vi "pumonarytesting_works.vi"() -> ()   [LabVIEW 2014]
uses:
  <vilib>/vision/NI_Vision_Development_Module.lvlib
  <instrlib>/KD Scientific 2XX Series/KD Scientific 2XX Series.lvlib
panel:
  in  "Number of Cycles":i32
  in  "Min Pressure":dbl
  in  "Max Pressure":dbl
  out "Status":T1
  in  "stop 2":bool
  out "Delivered Volume":dbl
  out "Units":string
  in  "Baud Rate (9600)":u32(ring)=9600 items=["300"=300, "1200"=1200, "2400"=2400, "4800"=4800, "9600"=9600]
  in  "Withdrawal Settings":T2={"Flow Rate (5)"=5.0, "Volume (10)"=10.0, "Volume Units (ml)"=enum."milliliters (ml)", "Rate Units (ml/min.)"=enum."milliliters per minute (ml/min.)"} {"Volume (10)" format="%#.3g"}
  in  "Diameter (8.75 mm)":dbl=8.75
  in  "Infusion Settings":T2={"Flow Rate (5)"=5.0, "Volume (10)"=10.0, "Volume Units (ml)"=enum."milliliters (ml)", "Rate Units (ml/min.)"=enum."milliliters per minute (ml/min.)"}
  in  "Address (0)":i32 format="%0.0f"
  in  "error in (no error)":errorcluster
  in  "VISA resource name":refnum<visa-resource-name>="COM1"
  in  "stop 4":bool
  in  "stop":bool
  out "Image":T3(plugin-control)
  out "Particle Measurements (Pixels) (Particle Analysis 1)":dbl[][](array[numeric]) format="%.2f"
  out "subarray":dbl[](array[numeric])
  out "The diameter":dbl[](array[numeric])
  in  "stop (F)":bool
  out "Data from Transducer":dynamicdata(graph) caption="Voltage from Transducer V"
  out "Voltage from pressure transducer":dbl[](array[numeric])
  out "Pressure mm Hg":dbl[](graph)
  in  "Calibration factor":dbl[](array[numeric])
  in  "Zero Error":dbl[](array[numeric])
  out "pressure mm Hg":dbl[](array[numeric])
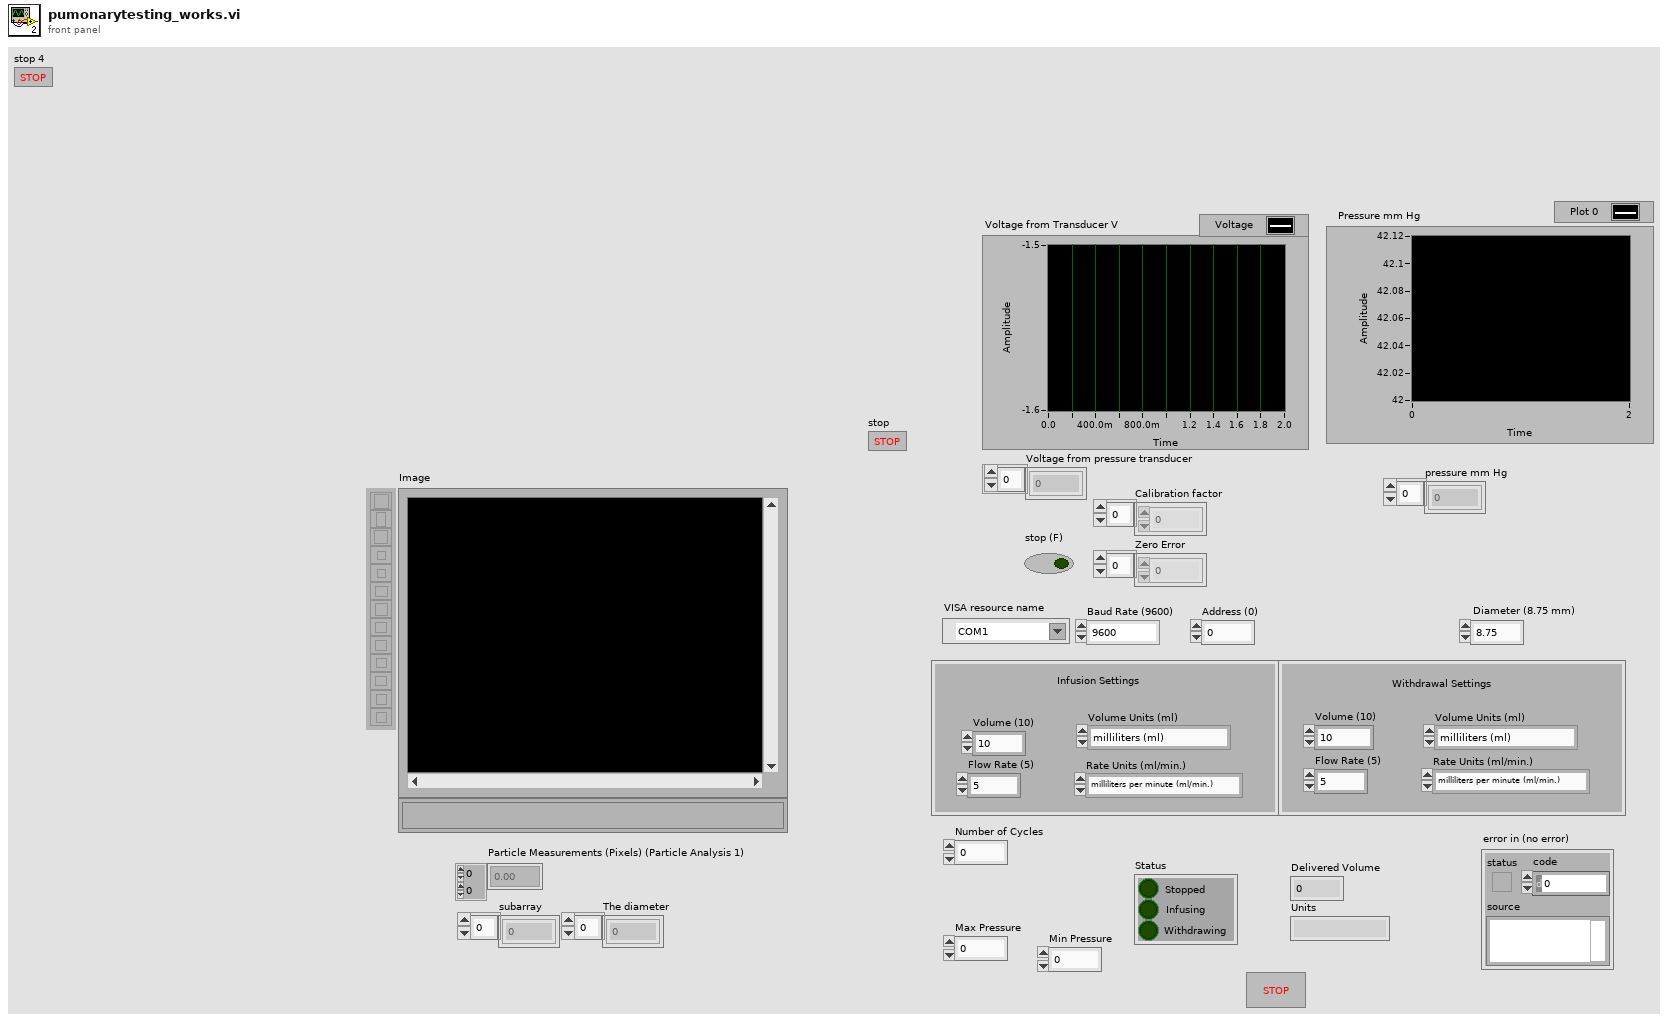
[diagram p1: front panel]
types:
  T1 = cluster{"Stopped":bool, "Infusing":bool, "Withdrawing":bool}
  T2 = cluster{"Flow Rate (5)":dbl, "Volume (10)":dbl, "Volume Units (ml)":enum16{"milliliters (ml)", "microliters (ul)"}, "Rate Units (ml/min.)":enum16{"milliliters per minute (ml/min.)", "milliliters per hour (ml/hr.)", "microliters per minute (ul/min.)", "microliters per hour (ul/hr.)"}}
  T3 = typedef "IMAQ Image.ctl" = refnum<image>
  T4 = typedef "Board Id" = u8
  T5 = typedef "ROI Descriptor" = cluster{"Global Rectangle":i32[], "Contours":cluster{"ID":enum32{"External", "Internal"}, "Type":u32, "Coordinates":i32[]}[]}
  T6 = enum16{"milliliters per minute (ml/min.)", "milliliters per hour (ml/hr.)", "microliters per minute (ul/min.)", "microliters per hour (ul/hr.)"}
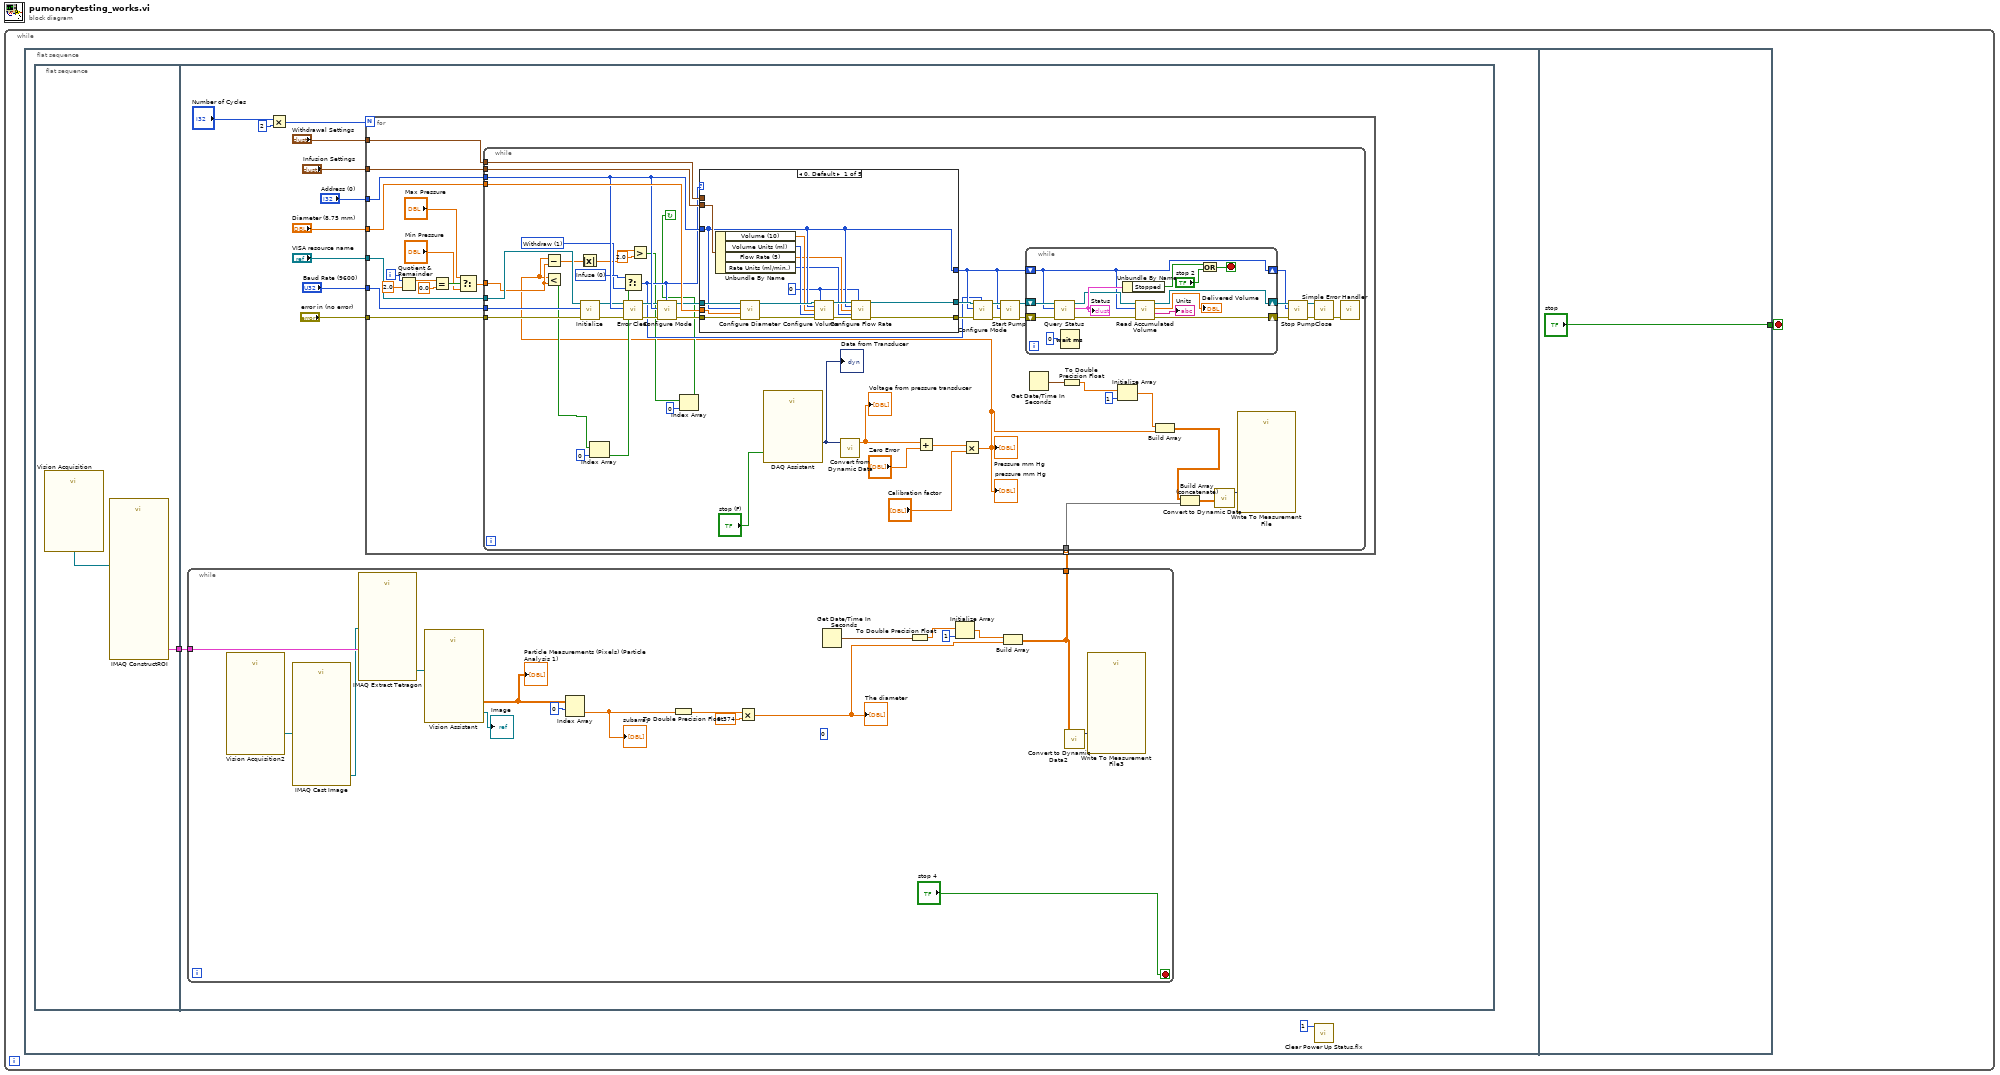
[diagram p0: block diagram]
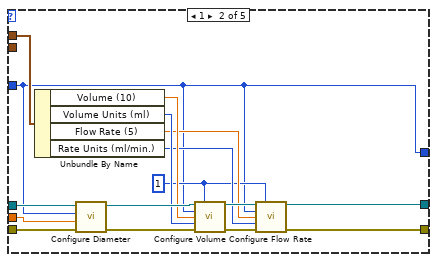
[diagram p2: hidden frame]
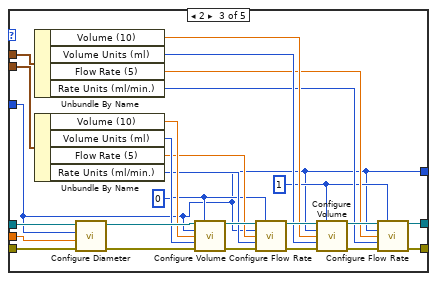
[diagram p3: hidden frame]
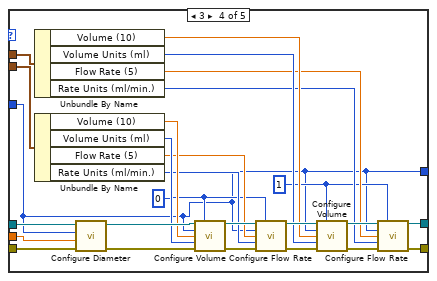
[diagram p4: hidden frame]
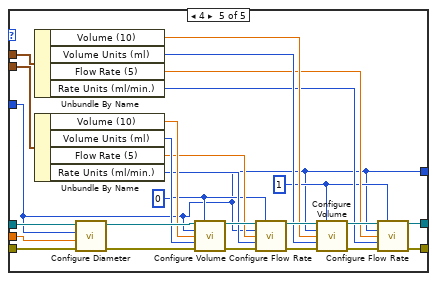
[diagram p5: hidden frame]
diagram:
  n1 = while {
    stop <- w1 stop-if-true
    n2 = flat-sequence {
      tunnel: ["stop"] -> w1
      frame #0 {
        n3 = flat-sequence {
          tunnel: [w4] -> w3
          tunnel: w3 -> [w17]
          frame #0 {
            n4 = call "Vision Acquisition"() -> ("Image Out"=w5:T3)  [unwired: 26 in, 1 out]
            n5 = call "IMAQ ConstructROI"("Image"=w5) -> ("ROI Descriptor Out"=w4:T5)  [unwired: 7 in, 3 out]
          }
          frame #1 {
            n6 = while {
              tunnel: w17 -> [w229]
              tunnel: [w212] -> w6
              stop <- "stop 4" stop-if-true
              (unwired) 0 ("index")
              n7 = call "Vision Acquisition2"() -> ("Image Out"=w220:T3)  [unwired: 25 in, 2 out]
              n8 = call "IMAQ Cast Image"("Image Src"=w220) -> ("Image Dst Out"=w226:T3)  [unwired: 9 in, 1 out]
              n9 = call-poly "IMAQ Extract Tetragon"("ROI Descriptor"=w229, "Image Src"=w226) -> ("Image Dst Out"=w227:T3)  [unwired: 8 in, 1 out]
              n10 = call "Vision Assistant"("Image In"=w227) -> ("Image Out"=→"Image":T3, "Particle Measurements (Pixels) (Particle Analysis 1)"=w225:dbl[][])  [unwired: 23 in, 2 out]
              "Particle Measurements (Pixels) (Particle Analysis 1)" <- w225
              n11 = Index Array(array=w225, index (row)=0) -> (element=w223:dbl[])  [unwired: 1 in]
              "subarray" <- w223
              n12 = To Double Precision Float(number=w223) -> (double precision float=w222:dbl[])
              n13 = Multiply(x=w222, y=0.374) -> (x*y=w214:dbl[])
              "The diameter" <- w214
              n14 = Get Date/Time In Seconds() -> (seconds since 1Jan1904=w218:timestamp)
              n15 = To Double Precision Float(number=w218) -> (double precision float=w217:dbl)
              n16 = Initialize Array(w217, 1 ("dimension size")) -> (w215:dbl[])
              n17 = Build Array(w215, w214) -> (w212:dbl[][])
              n18 = call "Convert to Dynamic Data2"("2D Array"=w212) -> ("Dynamic Data Type"=w213:dynamicdata)  [unwired: 3 in]
              n19 = call "Write To Measurement File3"("Signals"=w213) -> ()  [unwired: 16 in, 3 out]
            }
            n20 = Multiply(x="Number of Cycles", y=2) -> (x*y=w16:i32)
            n21 = for {
              N: w16 -> [_]
              tunnel: "VISA resource name" -> [w33]
              tunnel: "error in (no error)" -> [w32]
              tunnel: "Infusion Settings" -> [w31]
              tunnel: "Withdrawal Settings" -> [w30]
              tunnel: "Diameter (8.75 mm)" -> [w29]
              tunnel: "Baud Rate (9600)" -> [w28]
              tunnel: "Address (0)" -> [w27]
              tunnel: w6 -> [w18] mode=indexing
              i -> [w25]
              n22 = Quotient & Remainder(x=w25, y=2.0) -> (x-y*floor(x/y)=w23:dbl)  [unwired: 1 out]
              n23 = Equal?(x=w23, y=0.0) -> (x = y?=w22:bool)
              n24 = Select(t="Max Pressure", s=w22, f="Min Pressure") -> (s? t:f=w19:dbl)
              n25 = while {
                tunnel: w33 -> [w87]
                tunnel: w32 -> [w86]
                tunnel: w31 -> [w85]
                tunnel: w30 -> [w84]
                tunnel: w29 -> [w83]
                tunnel: w28 -> [w82]
                tunnel: w27 -> [w81]
                tunnel: w19 -> [w58]
                tunnel: w18 -> [w37]
                stop <- w43 continue-if-true
                w60 = u16 1 items=["Withdraw"=1]
                w61 = u16 0 items=["Infuse"] ("Mode (infuse)")
                n26 = call <instrlib>:"Initialize.vi"("error in (no error)"=w86, "Baud Rate (9600)"=w82, "VISA resource name"=w87) -> ("error out"=w63:errorcluster, "VISA resource name out"=w62:refnum<visa-resource-name>)  [unwired: 7 in]
                n27 = call <instrlib>:"Error Clear.vi"("error in (no error)"=w63, "Address (0)"=w81, "VISA resource name"=w62) -> ("error out"=w64:errorcluster, "VISA resource name out"=w65:refnum<visa-resource-name>)  [unwired: 6 in, 1 out]
                n28 = call "DAQ Assistant"("stop (T)"="stop (F)") -> ("data"=w49:dynamicdata)  [unwired: 16 in, 2 out]
                "Data from Transducer" <- w49
                n29 = call "Convert from Dynamic Data"("Dynamic Data Type"=w49) -> ("Array"=w52:dbl[])  [unwired: 3 in]
                "Voltage from pressure transducer" <- w52
                n30 = Add(x=w52, y="Zero Error") -> (x+y=w50:dbl[])
                n31 = Multiply(x=w50, y="Calibration factor") -> (x*y=w38:dbl[])
                "Pressure mm Hg" <- w38
                "pressure mm Hg" <- w38
                n32 = Subtract(x=w38, y=w58) -> (x-y=w57:dbl[])
                n33 = Less?(x=w38, y=w58) -> (x < y?=w48:bool[])
                n34 = Absolute Value(x=w57) -> (abs(x)=w56:dbl[])
                n35 = Index Array(array=w48, index=0) -> (element=w46:bool)
                n36 = Select(t=w61, s=w46, f=w60) -> (s? t:f=w59:u16)
                n37 = Greater?(x=w56, y=2.0) -> (0:w45:bool[])
                n38 = call <instrlib>:"Configure Mode.vi"("Mode (infuse)"=w59, "error in (no error)"=w64, "Address (0)"=w81, "VISA resource name"=w65) -> ("error out"=w67:errorcluster, "VISA resource name out"=w66:refnum<visa-resource-name>)  [unwired: 6 in]
                n39 = Index Array(array=w45, index=0) -> (element=w43:bool)
                n40 = case shown="0, Default" w59 {
                  tunnel: w85 -> [w97 _ w145 w171 w197]
                  tunnel: w84 -> [_ w119 w144 w170 w196]
                  tunnel: w66 -> [w103 w118 w143 w169 w195]
                  tunnel: w67 -> [w102 w114 w142 w168 w194]
                  tunnel: w83 -> [w96 w110 w125 w151 w177]
                  tunnel: [w95 w104 w120 w146 w172] -> w68
                  tunnel: w81 -> [w95 w104 w120 w146 w172]
                  tunnel: [w90 w115 w122 w148 w174] -> w72
                  tunnel: [w89 w111 w121 w147 w173] -> w71
                  frame 0, Default {
                    w88 = 0
                    n41 = Unbundle By Name(w97) -> ("Volume (10)"=w94:dbl, "Volume Units (ml)"=w93:enum16{"milliliters (ml)", "microliters (ul)"}, "Flow Rate (5)"=w92:dbl, "Rate Units (ml/min.)"=w91:T6)
                    n42 = call <instrlib>:"Configure Diameter.vi"("error in (no error)"=w102, "Diameter (8.75 mm)"=w96, "Address (0)"=w95, "VISA resource name"=w103) -> ("error out"=w100:errorcluster, "VISA resource name out"=w101:refnum<visa-resource-name>)  [unwired: 6 in]
                    n43 = call <instrlib>:"Configure Volume.vi"("VISA resource name"=w101, "Mode (infuse)"=w88, "Address (0)"=w95, "Volume (100)"=w94, "Units (0: milliliters)"=w93, "error in (no error)"=w100) -> ("VISA resource name out"=w99:refnum<visa-resource-name>, "error out"=w98:errorcluster)  [unwired: 8 in]
                    n44 = call <instrlib>:"Configure Flow Rate.vi"("VISA resource name"=w99, "Mode (infuse)"=w88, "Address (0)"=w95, "Flow Rate (5)"=w92, "Units (0: milliliters per minute)"=w91, "error in (no error)"=w98) -> ("VISA resource name out"=w90:refnum<visa-resource-name>, "error out"=w89:errorcluster)  [unwired: 8 in]
                  }
                  frame 1 {
                    w105 = 1
                    n45 = Unbundle By Name(w119) -> ("Volume (10)"=w109:dbl, "Volume Units (ml)"=w108:enum16{"milliliters (ml)", "microliters (ul)"}, "Flow Rate (5)"=w107:dbl, "Rate Units (ml/min.)"=w106:T6)
                    n46 = call <instrlib>:"Configure Diameter.vi"("error in (no error)"=w114, "Diameter (8.75 mm)"=w110, "Address (0)"=w104, "VISA resource name"=w118) -> ("error out"=w113:errorcluster, "VISA resource name out"=w117:refnum<visa-resource-name>)  [unwired: 6 in]
                    n47 = call <instrlib>:"Configure Volume.vi"("VISA resource name"=w117, "Mode (infuse)"=w105, "Address (0)"=w104, "Volume (100)"=w109, "Units (0: milliliters)"=w108, "error in (no error)"=w113) -> ("VISA resource name out"=w116:refnum<visa-resource-name>, "error out"=w112:errorcluster)  [unwired: 8 in]
                    n48 = call <instrlib>:"Configure Flow Rate.vi"("VISA resource name"=w116, "Mode (infuse)"=w105, "Address (0)"=w104, "Flow Rate (5)"=w107, "Units (0: milliliters per minute)"=w106, "error in (no error)"=w112) -> ("VISA resource name out"=w115:refnum<visa-resource-name>, "error out"=w111:errorcluster)  [unwired: 8 in]
                  }
                  frame 2 {
                    w123 = 1
                    w124 = 0
                    n49 = Unbundle By Name(w144) -> ("Volume (10)"=w129:dbl, "Volume Units (ml)"=w128:enum16{"milliliters (ml)", "microliters (ul)"}, "Flow Rate (5)"=w127:dbl, "Rate Units (ml/min.)"=w126:T6)
                    n50 = Unbundle By Name(w145) -> ("Volume (10)"=w133:dbl, "Volume Units (ml)"=w132:enum16{"milliliters (ml)", "microliters (ul)"}, "Flow Rate (5)"=w131:dbl, "Rate Units (ml/min.)"=w130:T6)
                    n51 = call <instrlib>:"Configure Diameter.vi"("error in (no error)"=w142, "Diameter (8.75 mm)"=w125, "Address (0)"=w120, "VISA resource name"=w143) -> ("error out"=w137:errorcluster, "VISA resource name out"=w141:refnum<visa-resource-name>)  [unwired: 6 in]
                    n52 = call <instrlib>:"Configure Volume.vi"("VISA resource name"=w141, "Mode (infuse)"=w124, "Address (0)"=w120, "Volume (100)"=w133, "Units (0: milliliters)"=w132, "error in (no error)"=w137) -> ("VISA resource name out"=w140:refnum<visa-resource-name>, "error out"=w136:errorcluster)  [unwired: 8 in]
                    n53 = call <instrlib>:"Configure Flow Rate.vi"("VISA resource name"=w140, "Mode (infuse)"=w124, "Address (0)"=w120, "Flow Rate (5)"=w131, "Units (0: milliliters per minute)"=w130, "error in (no error)"=w136) -> ("VISA resource name out"=w139:refnum<visa-resource-name>, "error out"=w135:errorcluster)  [unwired: 8 in]
                    n54 = call <instrlib>:"Configure Volume.vi"("VISA resource name"=w139, "Mode (infuse)"=w123, "Address (0)"=w120, "Volume (100)"=w129, "Units (0: milliliters)"=w128, "error in (no error)"=w135) -> ("VISA resource name out"=w138:refnum<visa-resource-name>, "error out"=w134:errorcluster)  [unwired: 8 in]
                    n55 = call <instrlib>:"Configure Flow Rate.vi"("VISA resource name"=w138, "Mode (infuse)"=w123, "Address (0)"=w120, "Flow Rate (5)"=w127, "Units (0: milliliters per minute)"=w126, "error in (no error)"=w134) -> ("VISA resource name out"=w122:refnum<visa-resource-name>, "error out"=w121:errorcluster)  [unwired: 8 in]
                  }
                  frame 3 {
                    w149 = 1
                    w150 = 0
                    n56 = Unbundle By Name(w170) -> ("Volume (10)"=w155:dbl, "Volume Units (ml)"=w154:enum16{"milliliters (ml)", "microliters (ul)"}, "Flow Rate (5)"=w153:dbl, "Rate Units (ml/min.)"=w152:T6)
                    n57 = Unbundle By Name(w171) -> ("Volume (10)"=w159:dbl, "Volume Units (ml)"=w158:enum16{"milliliters (ml)", "microliters (ul)"}, "Flow Rate (5)"=w157:dbl, "Rate Units (ml/min.)"=w156:T6)
                    n58 = call <instrlib>:"Configure Diameter.vi"("error in (no error)"=w168, "Diameter (8.75 mm)"=w151, "Address (0)"=w146, "VISA resource name"=w169) -> ("error out"=w163:errorcluster, "VISA resource name out"=w167:refnum<visa-resource-name>)  [unwired: 6 in]
                    n59 = call <instrlib>:"Configure Volume.vi"("VISA resource name"=w167, "Mode (infuse)"=w150, "Address (0)"=w146, "Volume (100)"=w159, "Units (0: milliliters)"=w158, "error in (no error)"=w163) -> ("VISA resource name out"=w166:refnum<visa-resource-name>, "error out"=w162:errorcluster)  [unwired: 8 in]
                    n60 = call <instrlib>:"Configure Flow Rate.vi"("VISA resource name"=w166, "Mode (infuse)"=w150, "Address (0)"=w146, "Flow Rate (5)"=w157, "Units (0: milliliters per minute)"=w156, "error in (no error)"=w162) -> ("VISA resource name out"=w165:refnum<visa-resource-name>, "error out"=w161:errorcluster)  [unwired: 8 in]
                    n61 = call <instrlib>:"Configure Volume.vi"("VISA resource name"=w165, "Mode (infuse)"=w149, "Address (0)"=w146, "Volume (100)"=w155, "Units (0: milliliters)"=w154, "error in (no error)"=w161) -> ("VISA resource name out"=w164:refnum<visa-resource-name>, "error out"=w160:errorcluster)  [unwired: 8 in]
                    n62 = call <instrlib>:"Configure Flow Rate.vi"("VISA resource name"=w164, "Mode (infuse)"=w149, "Address (0)"=w146, "Flow Rate (5)"=w153, "Units (0: milliliters per minute)"=w152, "error in (no error)"=w160) -> ("VISA resource name out"=w148:refnum<visa-resource-name>, "error out"=w147:errorcluster)  [unwired: 8 in]
                  }
                  frame 4 {
                    w175 = 1
                    w176 = 0
                    n63 = Unbundle By Name(w196) -> ("Volume (10)"=w181:dbl, "Volume Units (ml)"=w180:enum16{"milliliters (ml)", "microliters (ul)"}, "Flow Rate (5)"=w179:dbl, "Rate Units (ml/min.)"=w178:T6)
                    n64 = Unbundle By Name(w197) -> ("Volume (10)"=w185:dbl, "Volume Units (ml)"=w184:enum16{"milliliters (ml)", "microliters (ul)"}, "Flow Rate (5)"=w183:dbl, "Rate Units (ml/min.)"=w182:T6)
                    n65 = call <instrlib>:"Configure Diameter.vi"("error in (no error)"=w194, "Diameter (8.75 mm)"=w177, "Address (0)"=w172, "VISA resource name"=w195) -> ("error out"=w189:errorcluster, "VISA resource name out"=w193:refnum<visa-resource-name>)  [unwired: 6 in]
                    n66 = call <instrlib>:"Configure Volume.vi"("VISA resource name"=w193, "Mode (infuse)"=w176, "Address (0)"=w172, "Volume (100)"=w185, "Units (0: milliliters)"=w184, "error in (no error)"=w189) -> ("VISA resource name out"=w192:refnum<visa-resource-name>, "error out"=w188:errorcluster)  [unwired: 8 in]
                    n67 = call <instrlib>:"Configure Flow Rate.vi"("VISA resource name"=w192, "Mode (infuse)"=w176, "Address (0)"=w172, "Flow Rate (5)"=w183, "Units (0: milliliters per minute)"=w182, "error in (no error)"=w188) -> ("VISA resource name out"=w191:refnum<visa-resource-name>, "error out"=w187:errorcluster)  [unwired: 8 in]
                    n68 = call <instrlib>:"Configure Volume.vi"("VISA resource name"=w191, "Mode (infuse)"=w175, "Address (0)"=w172, "Volume (100)"=w181, "Units (0: milliliters)"=w180, "error in (no error)"=w187) -> ("VISA resource name out"=w190:refnum<visa-resource-name>, "error out"=w186:errorcluster)  [unwired: 8 in]
                    n69 = call <instrlib>:"Configure Flow Rate.vi"("VISA resource name"=w190, "Mode (infuse)"=w175, "Address (0)"=w172, "Flow Rate (5)"=w179, "Units (0: milliliters per minute)"=w178, "error in (no error)"=w186) -> ("VISA resource name out"=w174:refnum<visa-resource-name>, "error out"=w173:errorcluster)  [unwired: 8 in]
                  }
                }
                n70 = call <instrlib>:"Configure Mode.vi"("Mode (infuse)"=w59, "error in (no error)"=w71, "Address (0)"=w68, "VISA resource name"=w72) -> ("error out"=w69:errorcluster, "VISA resource name out"=w70:refnum<visa-resource-name>)  [unwired: 6 in]
                n71 = call <instrlib>:"Start Pump.vi"("error in (no error)"=w69, "Address (0)"=w68, "VISA resource name"=w70) -> ("error out"=w79:errorcluster, "VISA resource name out"=w80:refnum<visa-resource-name>)  [unwired: 7 in]
                n72 = while {
                  shift-right: [w200] -> w76
                  shift-left: w68 -> [w200]
                  shift-right: [w202] -> w78
                  shift-left: w80 -> [w208]
                  shift-right: [w201] -> w77
                  shift-left: w79 -> [w209]
                  stop <- w206 stop-if-true
                  n73 = call <instrlib>:"Query Status.vi"("error in (no error)"=w209, "Address (0)"=w200, "VISA resource name"=w208) -> ("error out"=w211:errorcluster, "Status"=w207:T1, "VISA resource name out"=w203:refnum<visa-resource-name>)  [unwired: 6 in]
                  "Status" <- w207
                  n74 = Wait (ms)(milliseconds to wait=u32 0) -> ()  [unwired: 1 out]
                  n75 = Unbundle By Name(w207) -> ("Stopped"=w205:bool)
                  n76 = call <instrlib>:"Read Accumulated Volume.vi"("error in (no error)"=w211, "Address (0)"=w200, "VISA resource name"=w203) -> ("error out"=w201:errorcluster, "Units"=→"Units":string, "Delivered Volume"=→"Delivered Volume":dbl, "VISA resource name out"=w202:refnum<visa-resource-name>)  [unwired: 5 in]
                  n77 = Or(x=w205, y="stop 2") -> (x .or. y?=w206:bool)
                }
                n78 = Get Date/Time In Seconds() -> (seconds since 1Jan1904=w42:timestamp)
                n79 = To Double Precision Float(number=w42) -> (double precision float=w41:dbl)
                n80 = Initialize Array(w41, 1 ("dimension size")) -> (w39:dbl[])
                n81 = Build Array(w39, w38) -> (w36:dbl[][])
                n82 = Build Array (concatenate)(w36, w37) -> (w35:dbl[][])
                n83 = call "Convert to Dynamic Data"("2D Array"=w35) -> ("Dynamic Data Type"=w34:dynamicdata)  [unwired: 3 in]
                n84 = call "Write To Measurement File"("Signals"=w34) -> ()  [unwired: 16 in, 3 out]
                n85 = call <instrlib>:"Stop Pump.vi"("error in (no error)"=w77, "Address (0)"=w76, "VISA resource name"=w78) -> ("error out"=w74:errorcluster, "VISA resource name out"=w73:refnum<visa-resource-name>)  [unwired: 7 in]
                n86 = call <instrlib>:"Close.vi"("error in (no error)"=w74, "VISA resource name"=w73) -> ("error out"=w75:errorcluster)  [unwired: 9 in]
                n87 = call <vilib>:"Simple Error Handler.vi"("error in (no error)"=w75) -> ()  [unwired: 4 in, 5 out]
              }
            }
          }
        }
        n88 = call <vilib>:"Clear Power Up Status.flx"("Board ID"=T4 1) -> ()  [unwired: 6 in, 2 out]
      }
      frame #1 {
      }
    }
  }
